vi "Runtime Test.vi"() -> ()   [LabVIEW 2021, in "Multiplexer tests.lvlib"]
doc: "This VI shows an example for how to test the Runtime functionality of the module. This will need to be modified according to module functionality."
uses:
  Multiplexer tests.lvlib
  execution/Multiplexer runtime.lvclass
  <vilib>/NI/Tag Bus/dictionary/data dictionary.lvclass/data dictionary.ctl
  <vilib>/NI/Tag Bus/dictionary/lookup polymorphs/locate double.vi
  <vilib>/NI/Tag Bus/table/data polymorphs/write many/write Doubles.vi
  <vilib>/NI/Tag Bus/dictionary/lookup polymorphs/locate Boolean.vi
  <vilib>/NI/Tag Bus/table/data polymorphs/write one/write Boolean.vi
  <vilib>/NI/Tag Bus/table/data polymorphs/read one/read Double.vi
  <vilib>/NI/Tag Bus/dictionary/search/find data index.vi
  <vilib>/NI/Tag Bus/dictionary/search/search string list.vi
  configuration/Multiplexer configuration.lvclass
  C:/Program Files (x86)/National Instruments/LabVIEW 2021/vi.lib/NI/Tag Bus Module Framework/module configuration/TBM module configuration.lvclass
  <vilib>/NI/Tag Bus/dictionary/tag not found.vi
  <vilib>/NI/Tag Bus/dictionary/data dictionary.lvclass
  <vilib>/NI/Tag Bus/table/data table.lvlib
panel:
  in  "Select":bool
  out "Processing Result":dbl
  in  "Processing Parameters":dbl[](array[numeric])
  out "error":errorcluster
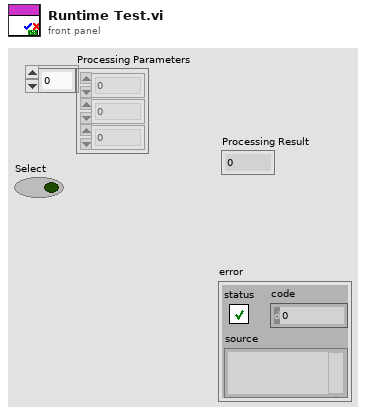
[diagram p1: front panel]
types:
  T1 = typedef "TBM channel.lvclass/data tables.ctl" = cluster{"input data":T2, "processing parameter":T2, "processing result":T2, "output data":T2}
  T2 = typedef "tag bus.lvlib/dictionary table pair.ctl" = cluster{"data dictionary":refnum<class "data dictionary.lvclass">, "data table":T3}
  T3 = typedef "tag bus.lvlib/data table.lvlib/data table.ctl" = cluster{"Double":dbl[], "Single":sgl[], "I64":i64[], "I32":i32[], "I16":i16[], "I8":i8[], "U64":u64[], "U32":u32[], "U16":u16[], "U8":u8[], "Boolean":bool[], "String":string[], "Array of Double":cluster{"DBL Array":dbl[]}[], "Array of Single":cluster{"SGL Array":sgl[]}[], "Array of I64":cluster{"I64 Array":i64[]}[], "Array of I32":cluster{"I32 Array":i32[]}[], "Array of I16":cluster{"I16 Array":i16[]}[], "Array of I8":cluster{"I8 Array":i8[]}[], "Array of U64":cluster{"U64 Array":u64[]}[], "Array of U32":cluster{"U32 Array":u32[]}[], "Array of U16":cluster{"U16 Array":u16[]}[], "Array of U8":cluster{"U8 Array":u8[]}[], "Array of Boolean":cluster{"Boolean Array":bool[]}[], "Array of String":cluster{"String Array":string[]}[]}
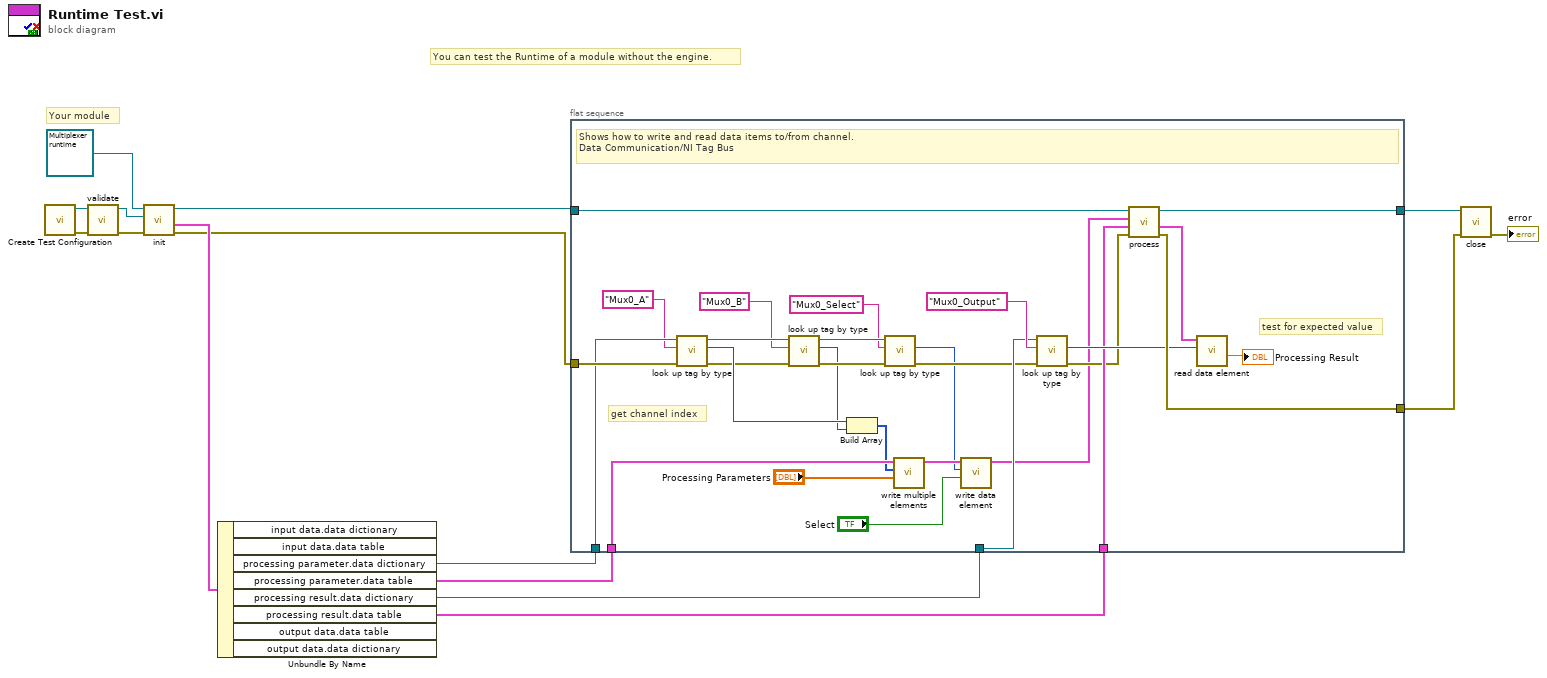
[diagram p0: block diagram]
diagram:
  # "You can test the Runtime of a module without the engine."
  # "Your module"
  n1 = call "Create Test Configuration.vi"() -> ("error out"=w11:errorcluster, "Module Configuration"=w12:refnum<class "Multiplexer configuration.lvclass">)  [unwired: 6 in, 4 out]
  n2 = call-dynamic "validate.vi"("error in"=w11, "Multiplexer configuration in"=w12) -> ("error out"=w14:errorcluster, "Multiplexer configuration out"=w13:refnum<class "Multiplexer configuration.lvclass">)  [unwired: 8 in]
  n3 = call-dynamic "init.vi"("error in"=w14, "TBM module configuration in"=w13, "Multiplexer runtime in"=refnum<class "Multiplexer runtime.lvclass"> refnum ("tag bus configurable plugin module")) -> ("error out"=w1:errorcluster, "data allocations"=w5:T1, "Multiplexer runtime out"=w4:refnum<class "Multiplexer runtime.lvclass">)  [unwired: 5 in, 1 out]
  n4 = Unbundle By Name(w5) -> ("processing parameter.data dictionary"=w10:refnum<class "data dictionary.lvclass">, "processing parameter.data table"=w9:T3, "processing result.data dictionary"=w7:refnum<class "data dictionary.lvclass">, "processing result.data table"=w6:T3)  [unwired: 4 out]
  n5 = flat-sequence {
    tunnel: w10 -> [w37]
    tunnel: w1 -> [w38]
    tunnel: w9 -> [w22]
    tunnel: [w44] -> w3
    tunnel: [w43] -> w2
    tunnel: w4 -> [w42]
    tunnel: w7 -> [w35]
    tunnel: w6 -> [w33]
    frame #0 {
      # "test for expected value"
      # "get channel index"
      # "Shows how to write and read data items to/from channel.\nData Communication/NI Tag Bus"
      n6 = call-poly <vilib>:"look up tag by type.vi"("error in"=w38, "name"="Mux0_A", "data dictionary in"=w37) -> ("error out"=w28:errorcluster, "index"=w39:i32, "data dictionary out"=w30:refnum<class "data dictionary.lvclass">)  [unwired: 6 in]
      n7 = call-poly <vilib>:"look up tag by type.vi"("error in"=w28, "name"="Mux0_B", "data dictionary in"=w30) -> ("error out"=w26:errorcluster, "index"=w24:i32, "data dictionary out"=w27:refnum<class "data dictionary.lvclass">)  [unwired: 6 in]
      n8 = Build Array(w39, w24) -> (w21:i32[])
      n9 = call-poly <vilib>:"look up tag by type.vi"("error in"=w26, "name"="Mux0_Select", "data dictionary in"=w27) -> ("error out"=w25:errorcluster, "index"=w18:i32)  [unwired: 6 in, 1 out]
      n10 = call-poly <vilib>:"write multiple elements.vi"("values"="Processing Parameters", "indices"=w21, "data table in"=w22) -> ("data table out"=w20:T3)  [unwired: 8 in]
      n11 = call-poly <vilib>:"write data element.vi"("value"="Select", "index"=w18, "data table in"=w20) -> ("data table out"=w19:T3)  [unwired: 8 in]
      n12 = call-poly <vilib>:"look up tag by type.vi"("error in"=w25, "name"="Mux0_Output", "data dictionary in"=w35) -> ("error out"=w32:errorcluster, "index"=w41:i32)  [unwired: 6 in, 1 out]
      n13 = call-dynamic "process.vi"("error in"=w32, "result allocation"=w33, "parameters"=w19, "module in"=w42) -> ("error out"=w43:errorcluster, "results"=w34:T3, "module out"=w44:refnum<class "Multiplexer runtime.lvclass">)  [unwired: 4 in, 1 out]
      n14 = call-poly <vilib>:"read data element.vi"("index"=w41, "data table in"=w34) -> ("value"=→"Processing Result":dbl)  [unwired: 8 in, 1 out]
    }
  }
  n15 = call-dynamic "close.vi"("error in"=w2, "Multiplexer runtime in"=w3) -> ("error out"=→"error":errorcluster)  [unwired: 9 in]
